vi "realTimeDisplay_MR1.vi"() -> ()   [LabVIEW 2016]
uses:
  <userlib>/RSA_API/RSA_API.lvlib
panel:
  in  "Done":bool
  in  "Cluster":T1 {"verticalUnit" items=["SpectrumVerticalUnit_dBm", "SpectrumVerticalUnit_Watt", "SpectrumVerticalUnit_Volt", "SpectrumVerticalUnit_Amp", "SpectrumVerticalUnit_dBmV"]; "window" items=["SpectrumWindow_Kaiser", "SpectrumWindow_Mil6dB", "SpectrumWindow_BlackmanHarris", "SpectrumWindow_Rectangle", "SpectrumWindow_FlatTop", "SpectrumWindow_Hann"]}
  in  "center freq":dbl
  in  "refLevel in":dbl
  in  "Trace number":u32(ring) items=["SpectrumTrace1", "SpectrumTrace2", "SpectrumTrace3"]
  out "traceData out":sgl[](graph)
  out "outTracePoints out":i32
  out "Trace Ready":bool
  out "enable out":bool
  out "refLevel out":dbl
  out "cf out":dbl
  in  "deviceID":i32
  out "deviceType out":string
  out "deviceSerial out":string
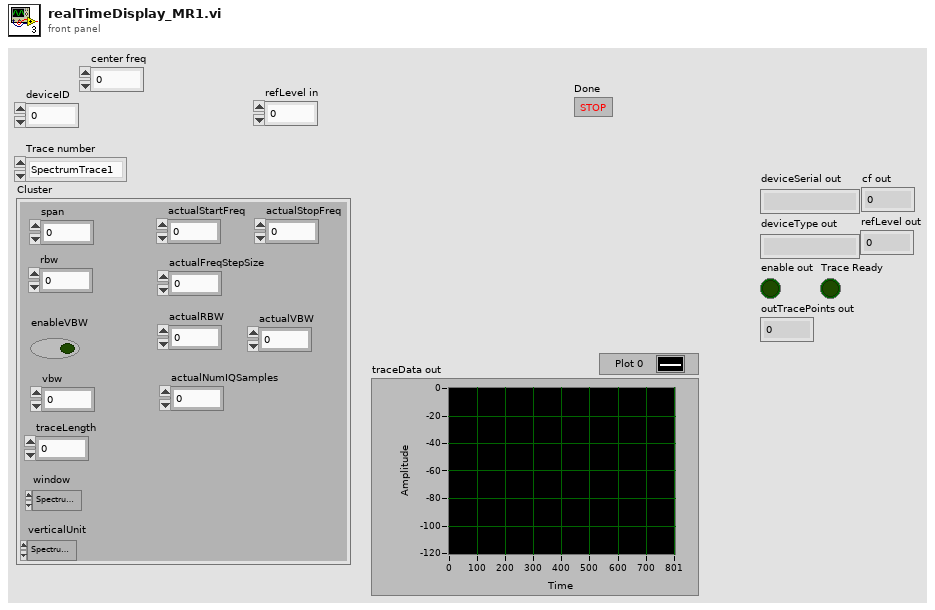
[diagram p1: front panel]
types:
  T1 = cluster{"span":dbl, "rbw":dbl, "enableVBW":bool, "vbw":dbl, "traceLength":i32, "window":u32, "verticalUnit":u32, "actualStartFreq":dbl, "actualStopFreq":dbl, "actualFreqStepSize":dbl, "actualRBW":dbl, "actualVBW":dbl, "actualNumIQSamples":i32}
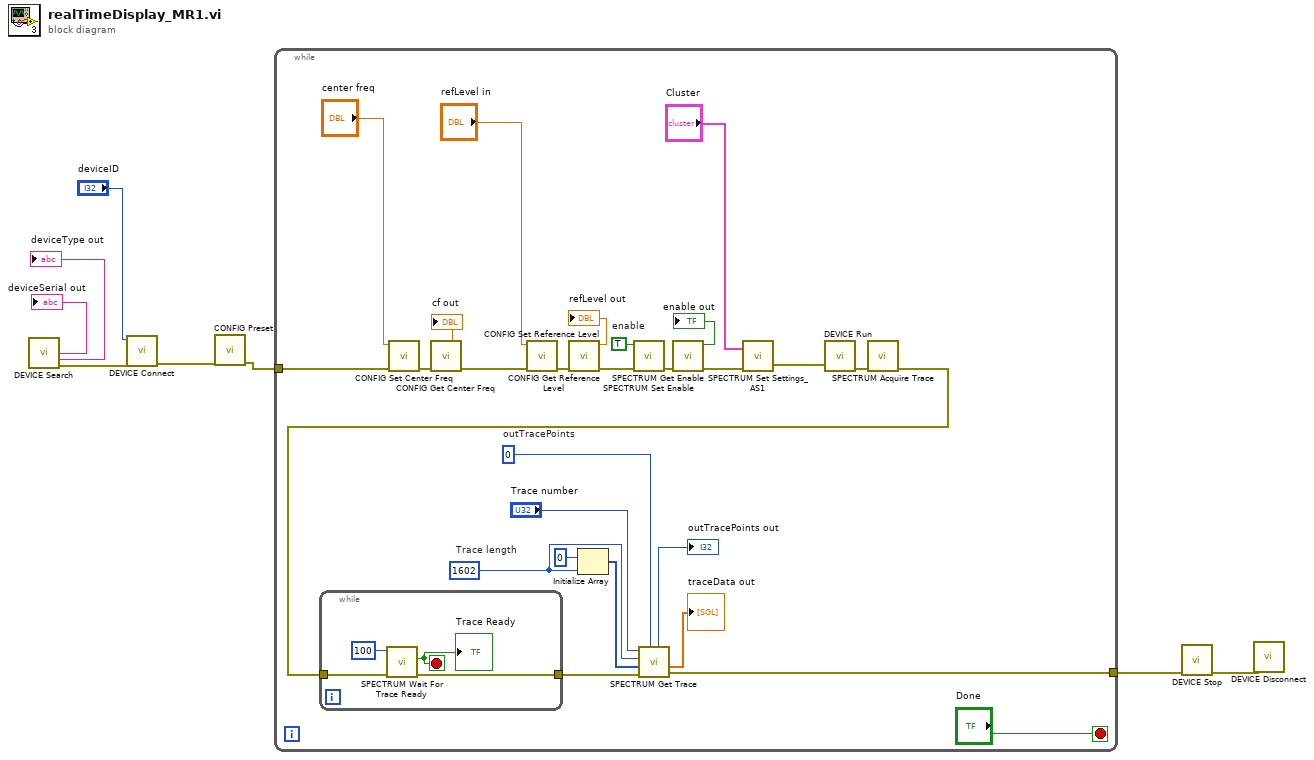
[diagram p0: block diagram]
diagram:
  n1 = call <userlib>:"DEVICE Search.vi"() -> ("deviceSerial out"=→"deviceSerial out":string, "deviceType out"=→"deviceType out":string, "error out"=w5:errorcluster)  [unwired: 10 in, 3 out]
  n2 = call <userlib>:"DEVICE Connect.vi"("error in (no error)"=w5, "deviceID"="deviceID") -> ("error out"=w4:errorcluster)  [unwired: 8 in, 1 out]
  n3 = call <userlib>:"CONFIG Preset.vi"("error in (no error)"=w4) -> ("error out"=w3:errorcluster)  [unwired: 9 in, 1 out]
  n4 = while {
    tunnel: w3 -> [w11]
    tunnel: [w9] -> w1
    stop <- "Done" stop-if-true
    w29 = TRUE  # enable
    w21 = 1602  # Trace length
    w22 = 0  # outTracePoints
    n5 = call <userlib>:"CONFIG Set Center Freq.vi"("error in (no error)"=w11, "cf"="center freq") -> ("error out"=w16:errorcluster)  [unwired: 8 in, 1 out]
    n6 = call <userlib>:"CONFIG Get Center Freq.vi"("error in (no error)"=w16) -> ("error out"=w35:errorcluster, "cf out"=→"cf out":dbl)  [unwired: 8 in, 1 out]
    n7 = call <userlib>:"CONFIG Set Reference Level.vi"("error in (no error)"=w35, "refLevel"="refLevel in") -> ("error out"=w34:errorcluster)  [unwired: 8 in, 1 out]
    n8 = call <userlib>:"CONFIG Get Reference Level.vi"("error in (no error)"=w34) -> ("error out"=w30:errorcluster, "refLevel out"=→"refLevel out":dbl)  [unwired: 8 in, 1 out]
    n9 = Initialize Array(0 ("element"), w21) -> (w19:i32[])
    n10 = call <userlib>:"SPECTRUM Set Enable.vi"("error in (no error)"=w30, "enable"=w29) -> ("error out"=w28:errorcluster)  [unwired: 8 in, 1 out]
    n11 = call <userlib>:"SPECTRUM Get Enable.vi"("error in (no error)"=w28) -> ("error out"=w14:errorcluster, "enable out"=→"enable out":bool)  [unwired: 8 in, 1 out]
    n12 = call "SPECTRUM Set Settings_AS1.vi"("error in (no error)"=w14, "Cluster"="Cluster") -> ("error out"=w13:errorcluster)  [unwired: 1 out]
    n13 = call <userlib>:"DEVICE Run.vi"("error in (no error)"=w13) -> ("error out"=w26:errorcluster)  [unwired: 9 in, 1 out]
    n14 = call <userlib>:"SPECTRUM Acquire Trace.vi"("error in (no error)"=w26) -> ("error out"=w25:errorcluster)  [unwired: 9 in, 1 out]
    n15 = while {
      tunnel: w25 -> [w37]
      tunnel: [w36] -> w24
      stop <- w38 stop-if-true
      n16 = call <userlib>:"SPECTRUM Wait For Trace Ready.vi"("error in (no error)"=w37, "timeoutMsec"=100) -> ("error out"=w36:errorcluster, "ready out"=w38:bool)  [unwired: 7 in, 1 out]
      "Trace Ready" <- w38
    }
    n17 = call <userlib>:"SPECTRUM Get Trace.vi"("outTracePoints"=w22, "error in (no error)"=w24, "traceData"=w19, "maxTracePoints"=w21, "trace"="Trace number") -> ("error out"=w9:errorcluster, "traceData out"=→"traceData out":sgl[], "outTracePoints out"=→"outTracePoints out":i32)  [unwired: 3 in, 1 out]
  }
  n18 = call <userlib>:"DEVICE Stop.vi"("error in (no error)"=w1) -> ("error out"=w2:errorcluster)  [unwired: 9 in, 1 out]
  n19 = call <userlib>:"DEVICE Disconnect.vi"("error in (no error)"=w2) -> ()  [unwired: 9 in, 2 out]
